vi "Plot Helper (Percentage).vi"(5 "error b percentage":dbl[](array[numeric]), 7 "error a percentage":dbl[](array[numeric]), 8 "error in (no error)":errorcluster, 9 "y vector":dbl[](array[numeric]), 10 "x vector":dbl[](array[numeric]), 11 "2D Plot Class Obj Array in":refnum<class "2D Plot Datatype.lvclass">[](array[class])) -> (0 "error out":errorcluster, 3 "2D Plot Class Obj Array out":refnum<class "2D Plot Datatype.lvclass">[](array[class]))   [LabVIEW 2020, in "2D Error Bar Datatype.lvclass"]
doc: "Graphs a plot that displays the percentage or vector of error at each point above and below the line graph. Multiple references to this VI generate multiple plots on the same graph."
uses:
  <vilib>/Math Plots/2D Math Plots/2D Error Bar/2D Error Bar Datatype/2D Error Bar Datatype.lvclass
  <vilib>/Math Plots/2D Math Plots/2D Plot/2D Plot Datatype/2D Plot Datatype.lvclass
  e:/builds/penguin/labview/branches/2020/dev/dist/vi.lib/Math Plots/2D Math Plots/2D Plot/2D Plot Datatype/2D Plot Datatype.lvclass
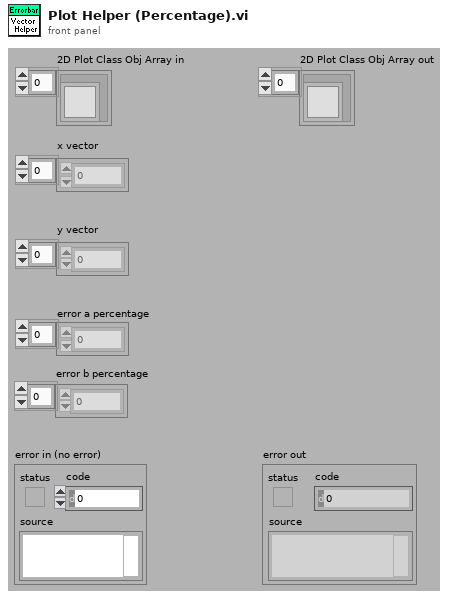
[diagram p1: front panel]
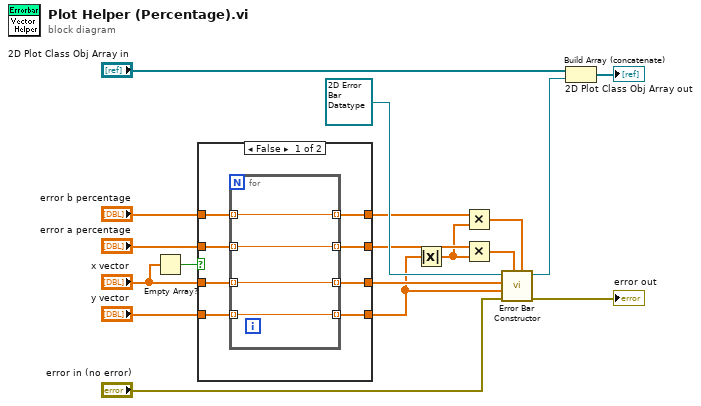
[diagram p0: block diagram]
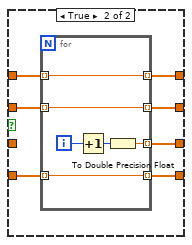
[diagram p2: hidden frame]
diagram:
  n1 = Empty Array?(array="x vector") -> (empty?=w11:bool)
  n2 = case shown="False" w11 {
    tunnel: "y vector" -> [w26 w36]
    tunnel: [w25 w33] -> w4
    tunnel: [w24 w34] -> w8
    tunnel: [w23 w35] -> w6
    tunnel: "error a percentage" -> [w22 w37]
    tunnel: "x vector" -> [w21 _]
    tunnel: [w20 w32] -> w5
    tunnel: "error b percentage" -> [w19 w31]
    frame False {
      n3 = for {
        tunnel: [w30] -> w24 mode=indexing
        tunnel: w21 -> [w30] mode=indexing
        tunnel: [w29] -> w25 mode=indexing
        tunnel: w26 -> [w29] mode=indexing
        tunnel: [w28] -> w23 mode=indexing
        tunnel: w22 -> [w28] mode=indexing
        tunnel: [w27] -> w20 mode=indexing
        tunnel: w19 -> [w27] mode=indexing
      }
    }
    frame True {
      n4 = for {
        tunnel: [w40] -> w34 mode=indexing
        tunnel: [w43] -> w33 mode=indexing
        tunnel: w36 -> [w43] mode=indexing
        tunnel: [w42] -> w35 mode=indexing
        tunnel: w37 -> [w42] mode=indexing
        tunnel: [w38] -> w32 mode=indexing
        tunnel: w31 -> [w38] mode=indexing
        i -> [w41]
        n5 = Increment(x=w41) -> (x+1=w39:i32)
        n6 = To Double Precision Float(number=w39) -> (double precision float=w40:dbl)
      }
    }
  }
  n7 = Absolute Value(x=w4) -> (abs(x)=w1:dbl[])
  n8 = Multiply(x=w5, y=w1) -> (x*y=w3:dbl[])
  n9 = Multiply(x=w6, y=w1) -> (x*y=w2:dbl[])
  n10 = call <vilib>:"Error Bar Constructor.vi"("error b vector"=w3, "error a vector"=w2, "error in (no error)"="error in (no error)", "y vector"=w4, "x vector"=w8, "2D Error Bar Datatype.lvclass in"=refnum<class "2D Error Bar Datatype.lvclass"> refnum ("3D Quiver Datatype.lvclass in")) -> ("error out"=→"error out":errorcluster, "2D Error Bar Datatype.lvclass out"=w17:refnum<class "2D Error Bar Datatype.lvclass">)  [unwired: 1 in, 3 out]
  n11 = Build Array (concatenate)("2D Plot Class Obj Array in", w17) -> (→"2D Plot Class Obj Array out":refnum<class "2D Plot Datatype.lvclass">[])
